vi "XY Graph setup.vi"(8 "Slide Refnum":refnum<vi>, 9 "Array - String":string[](array[string]), 10 "XYGraph Refnum":refnum<vi>) -> (1 "Total Bounds Rect":T2)   [LabVIEW 2016]
uses:
  <vilib>/Utility/miscctls.llb/LVRectTypeDef.ctl
  <vilib>/picture/picture.llb/Draw True-Color Pixmap.vi
panel:
  out "error out 2":errorcluster
  out "Current plot color":u32(colorbox)
  out "current plot":u32
  out "Active PLOT":u32[](array[numeric])
  out "Text Color":u32[](array[colorbox])
  out "Plot before":u32[](array[colorbox])
  out "error out":errorcluster
  out "new picture":picture
  out "size(s) 2":i32
  out "abs(x)":i32
  out "x-y":i32
  out "output cluster":T1
  out "size(s)":i32
  out "String":string
  out "Plot Area Bounds":T2
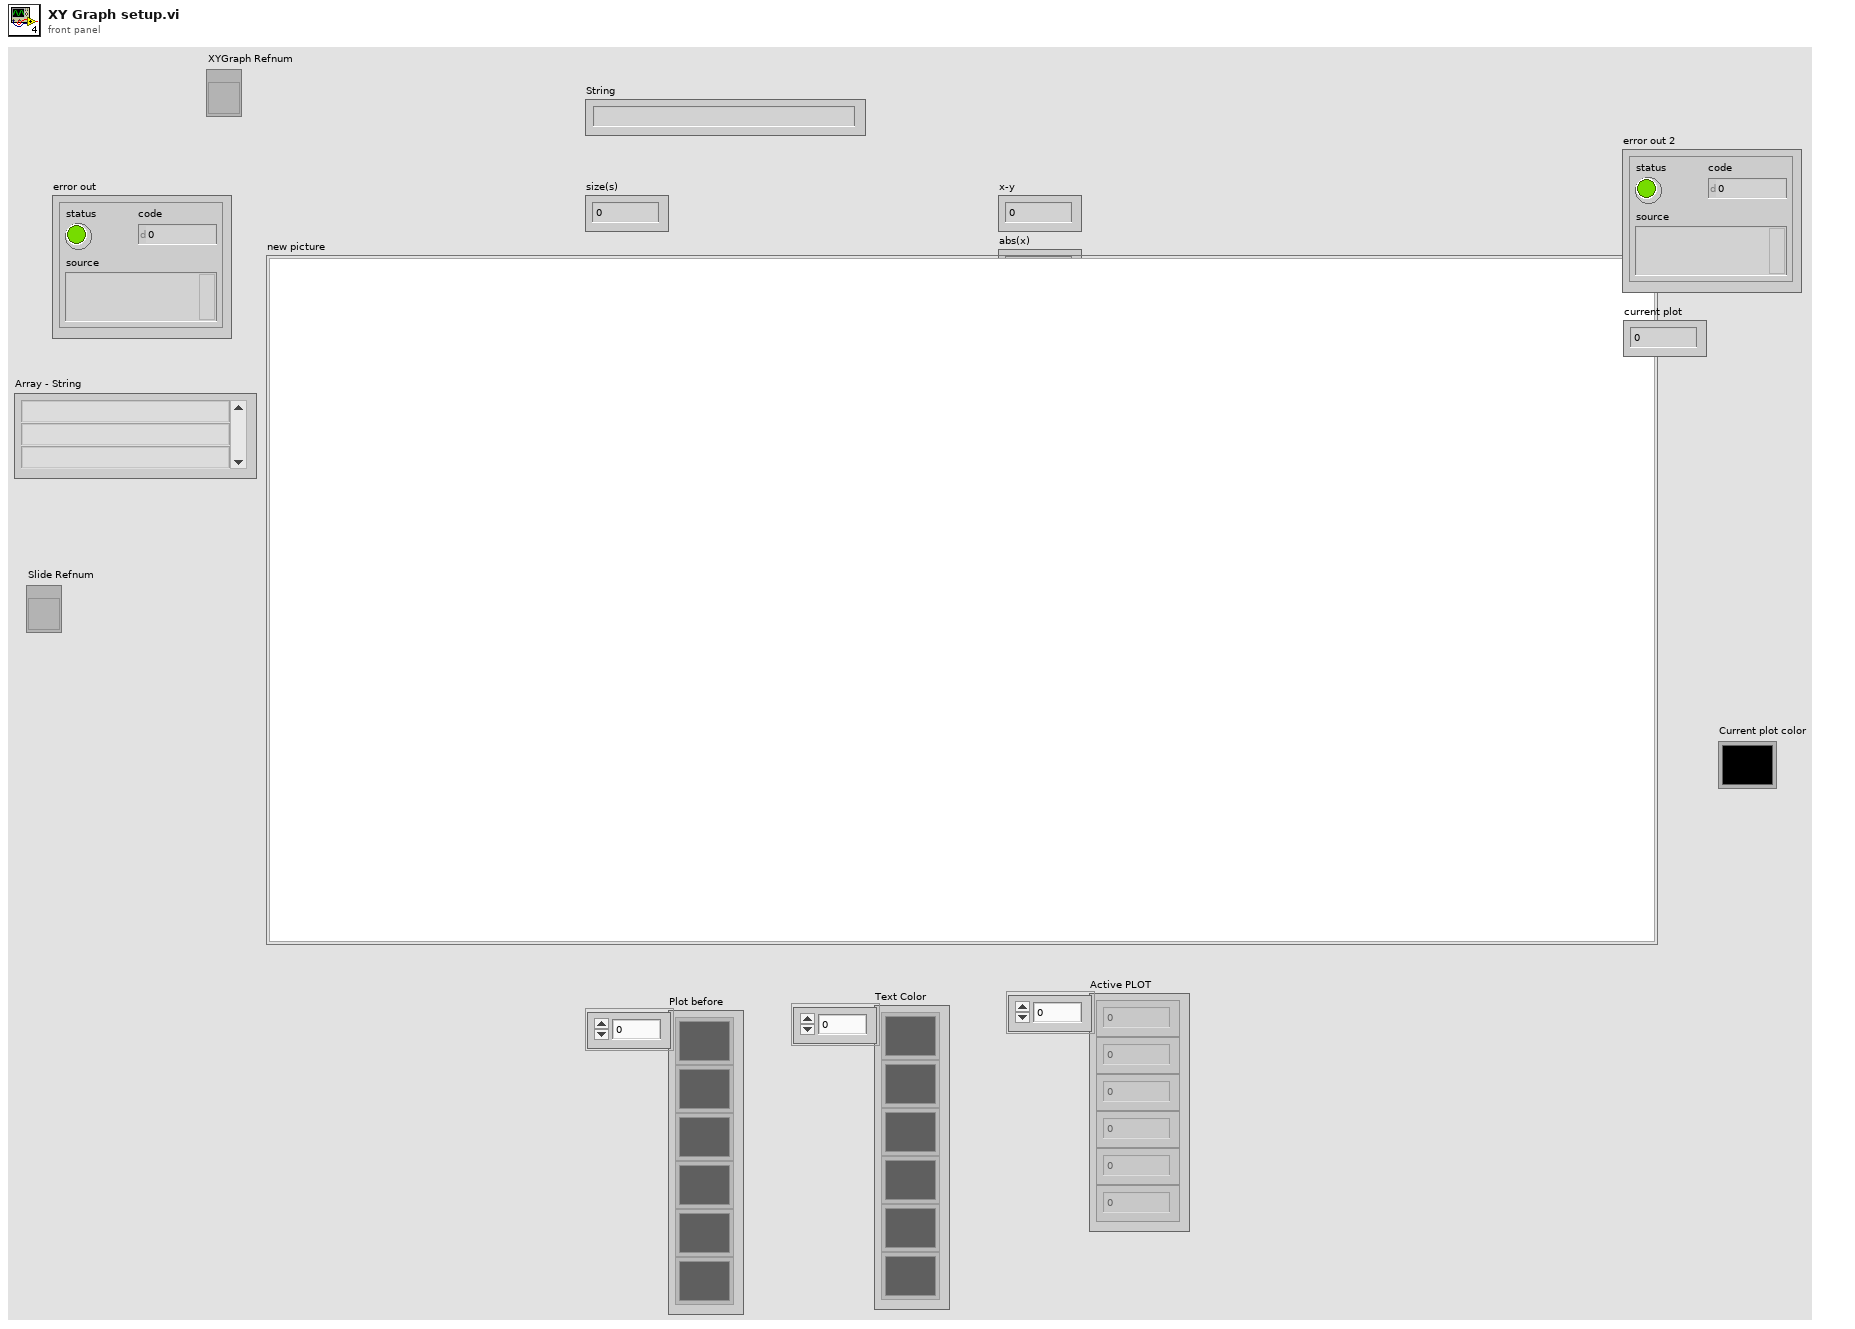
[diagram p1: front panel]
types:
  T1 = cluster{"Numeric Control":i32, "Numeric Control":i32}
  T2 = typedef "LVRectTypeDef.ctl" = cluster{"Left":i16, "Top":i16, "Right":i16, "Bottom":i16}
  T3 = typedef "LVPoint32TypeDef.ctl" = cluster{"Horizontal":i32, "Vertical":i32}
  T4 = cluster{"left":i16, "top":i16, "right":i16, "bottom":i16}
  T5 = typedef "imagedata.ctl" = cluster{"image type":i32, "image depth":i32, "image":u8[], "mask":u8[], "colors":u32[], "Rectangle":cluster{"left":i16, "top":i16, "right":i16, "bottom":i16}}
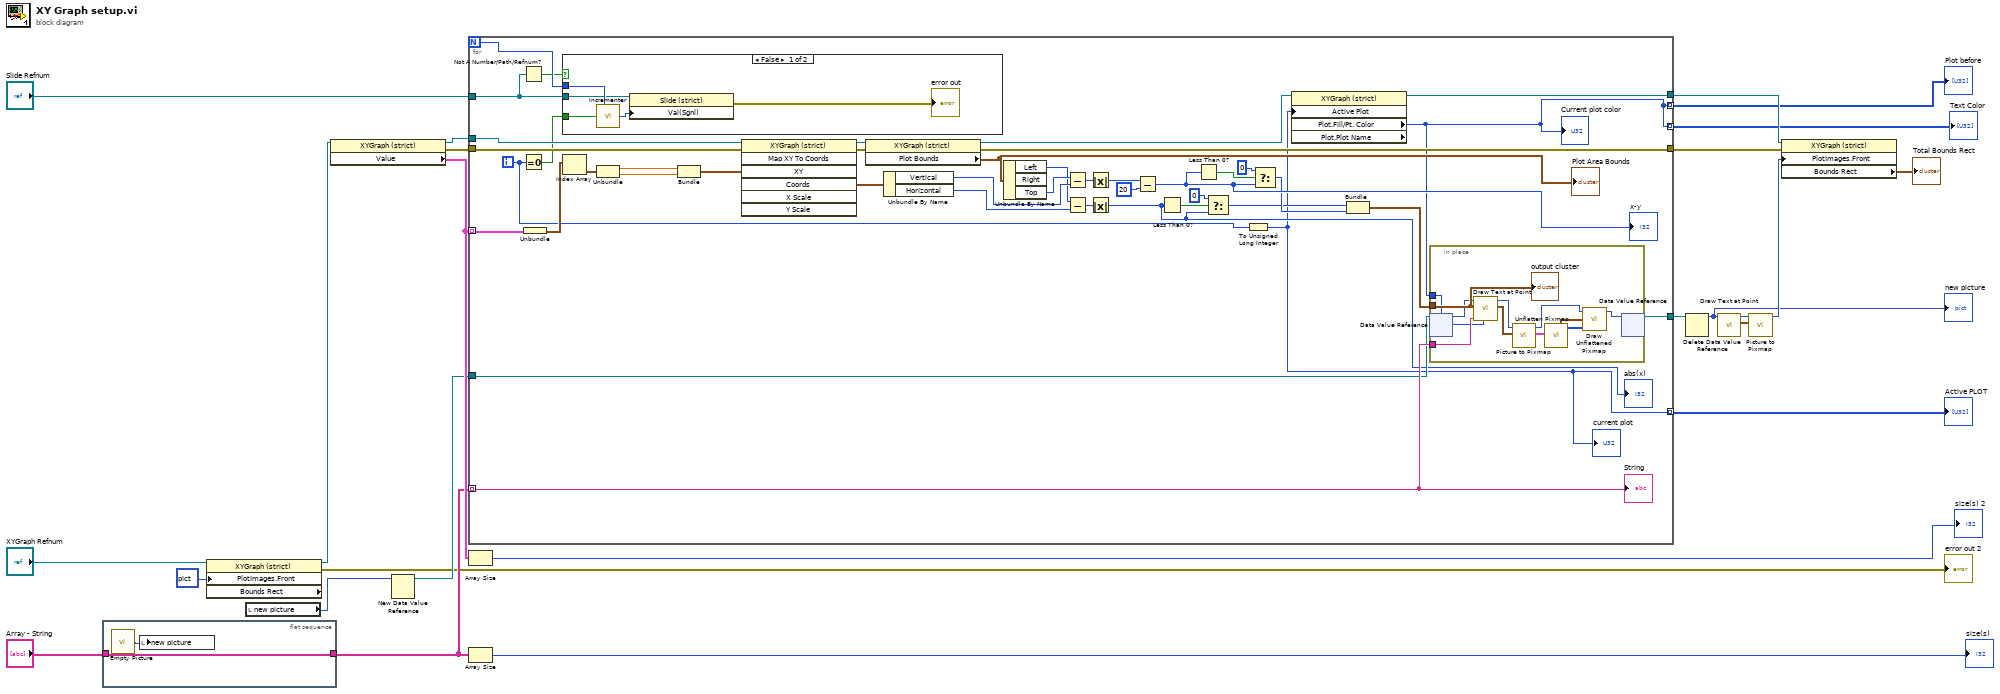
[diagram p0: block diagram]
diagram:
  n1 = flat-sequence {
    tunnel: [w26] -> w9
    tunnel: "Array - String" -> [w26]
    frame #0 {
      n2 = call "Empty Picture"() -> ("empty picture"=w27:picture)
      n3 = local write "new picture"(w27) -> ()
    }
  }
  n4 = property on="Property Node" class="XYGraph (strict)" props=["PlotImages.Front", "Bounds Rect"](reference="XYGraph Refnum", "PlotImages.Front"=picture data[5B] ("Plot Images:Front")) -> (reference out=w14:refnum<vi>, error out=→"error out 2":errorcluster)  [unwired: 1 in, 1 out]
  n5 = local read "new picture"() -> (w8:picture)
  n6 = property class="XYGraph (strict)"(reference=w14) -> (reference out=w13:refnum<vi>, error out=w21:errorcluster, "Value"=w25:cluster{cluster{dbl, "index":dbl}[]}[])  [unwired: 1 in]
  n7 = New Data Value Reference(data value=w8) -> (data value reference=w7:refnum<data-value>)  [unwired: 1 in, 1 out]
  n8 = for {
    N -> [w62]
    tunnel: w25 -> [w68] mode=indexing
    tunnel: w9 -> [w64] mode=indexing
    tunnel: "Slide Refnum" -> [w34]
    tunnel: w13 -> [w69]
    tunnel: [w28] -> w22
    tunnel: w21 -> [w65]
    tunnel: [w66] -> w20
    tunnel: w7 -> [w36]
    tunnel: [w35] -> w6
    tunnel: [w29] -> w4 mode=indexing
    tunnel: [w29] -> w3 mode=indexing
    tunnel: [w30] -> w2 mode=indexing
    i -> [w32]
    n9 = Not A Number/Path/Refnum?(number/path/refnum=w34) -> (NaN/Path/Refnum?=w33:bool)
    n10 = Equal To 0?(x=w32) -> (x = 0?=w63:bool)
    n11 = Unbundle(w68) -> (w38:cluster{dbl, "index":dbl}[])
    n12 = case shown="False" w33 {
      tunnel: w63 -> [w74 _]
      tunnel: w62 -> [w73 _]
      tunnel: w34 -> [w71 _]
      frame False {
        n13 = call "Incrementer.vi"("N"=w73, "reset"=w74) -> ("Count"=w72:i32)  [unwired: 13 in]
        n14 = property class="Slide (strict)"(reference=w71, "Val(Sgnl)"=w72) -> (error out=→"error out":errorcluster)  [unwired: 1 in, 1 out]
      }
      frame True {
      }
    }
    n15 = Index Array(array=w38) -> (element=w37:cluster{dbl, "index":dbl})  [unwired: 1 in]
    n16 = Unbundle(w37) -> (w50:dbl, "index"=w51:dbl)
    n17 = Bundle(w50, "index"=w51) -> (w59:cluster{dbl, "index":dbl})  [unwired: 1 in]
    n18 = invoke class="XYGraph (strict)" method="Map XY To Coords"(reference=w69, error in=w65, "XY"=w59) -> (reference out=w67:refnum<vi>, error out=w52:errorcluster, "Coords"=w60:T3)  [unwired: 4 in, 4 out]
    n19 = property on="Property Node" class="XYGraph (strict)"(reference=w67, error in=w52) -> (reference out=w46:refnum<vi>, error out=w66:errorcluster, "Plot Bounds"=w61:T2)
    "Plot Area Bounds" <- w61
    n20 = Unbundle By Name(w60) -> ("Vertical"=w53:i32, "Horizontal"=w48:i32)
    n21 = Unbundle By Name(w61) -> ("Left"=w49:i16, "Top"=w58:i16)  [unwired: 1 out]
    n22 = Subtract(x=w58, y=w53) -> (x-y=w57:i32)
    n23 = Subtract(x=w49, y=w48) -> (x-y=w47:i32)
    n24 = Absolute Value(x=w57) -> (abs(x)=w56:i32)
    n25 = Absolute Value(x=w47) -> (abs(x)=w31:i32)
    "abs(x)" <- w31
    n26 = Subtract(x=w56, y=20) -> (x-y=w44:i32)
    "x-y" <- w44
    n27 = Less Than 0?(x=w31) -> (x < 0?=w41:bool)
    n28 = Less Than 0?(x=w44) -> (x < 0?=w45:bool)
    n29 = Select(t=0, s=w41, f=w31) -> (s? t:f=w39:i32)
    n30 = To Unsigned Long Integer(number=w32) -> (unsigned 32bit integer=w30:u32)
    "current plot" <- w30
    n31 = Select(t=0, s=w45, f=w44) -> (s? t:f=w42:i32)
    n32 = property on="Property Node" class="XYGraph (strict)" props=["Active Plot", "Plot", "Fill/Pt. Color", "Plot", "Plot Name"](reference=w46, "Active Plot"=w30) -> (reference out=w28:refnum<vi>, "Plot.Fill/Pt. Color"=w29:u32)  [unwired: 1 in, 2 out]
    "Current plot color" <- w29
    n33 = Bundle("t"=w39, "t"=w42) -> (w55:cluster{"t":i32, "t":i32})  [unwired: 1 in]
    n34 = in-place {
      in-place-border: w64 -> [w85]
      in-place-border: w55 -> [w84]
      in-place-border: w29 -> [w83]
      n35 = in-place-dvr #1(w36) -> (w76:picture)  [unwired: 1 out]
      n36 = call <vilib>:"Draw Text at Point.vi"("text color(black)"=w83, "text"=w85, "origin"=w84, "picture"=w76) -> ("text rect"=w80:T4, "new picture"=w81:picture)  [unwired: 6 in]
      n37 = call <vilib>:"Picture to Pixmap.vi"("rect"=w80, "picture"=w81) -> ("image data"=w82:T5, "new picture"=w77:picture)  [unwired: 8 in]
      n38 = call <vilib>:"Unflatten Pixmap.vi"("image data"=w82) -> ("24-bit pixmap"=w78:u32[][], "top left"=w79:cluster{"x":i16, "y":i16})  [unwired: 4 in, 5 out]
      n39 = call-poly <vilib>:"Draw Unflattened Pixmap.vi"("picture"=w77, "top left point(0, 0)"=w79, "data (RGB format)"=w78) -> ("new picture"=w75:picture)  [unwired: 6 in]
      n40 = in-place-dvr #1(w75) -> (w35:refnum<data-value>)  [unwired: 1 out]
      "output cluster" <- w84
    }
    "String" <- w64
  }
  "Plot before" <- w4
  "Text Color" <- w3
  "Active PLOT" <- w2
  n41 = Array Size(array=w25) -> (size(s)=→"size(s) 2":i32)
  n42 = Array Size(array=w9) -> (size(s)=→"size(s)":i32)
  n43 = Delete Data Value Reference(data value reference=w6) -> (data value=w5:picture)  [unwired: 1 in, 1 out]
  "new picture" <- w5
  n44 = call <vilib>:"Draw Text at Point.vi"("picture"=w5) -> ("text rect"=w18:T4, "new picture"=w17:picture)  [unwired: 9 in]
  n45 = call <vilib>:"Picture to Pixmap.vi"("rect"=w18, "picture"=w17) -> ("new picture"=w19:picture)  [unwired: 8 in, 1 out]
  n46 = property on="Property Node" class="XYGraph (strict)"(reference=w22, error in=w20, "PlotImages.Front"=w19) -> ("Bounds Rect"=→"Total Bounds Rect":T2)  [unwired: 2 out]
